vi "XLP80_EA_ReadStatus_Stack.vi"(8 "err in":errorcluster, 11 "Device information":string[](array[string])=["ASRL1::INSTR", "EL 3160-60 A", "000", "///", "1", "160", "60", "400", "10", "400"]) -> (0 "err out":errorcluster, 2 "Remote ON":bool, 3 "Device information IN":string[](array[string])=["ASRL1::INSTR", "EL 3160-60 A", "000", "///", "1", "160", "60", "400", "10", "400"])   [LabVIEW 2021]
uses:
  XLP80_EA_TDefsCluster_EA Feedback.ctl
  XLP80_EA_Globals.vi
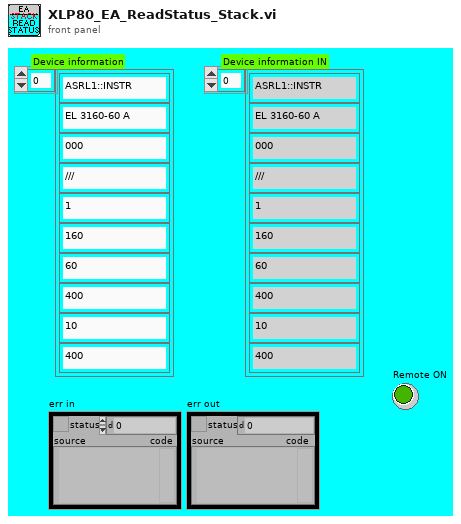
[diagram p1: front panel]
types:
  T1 = typedef "XLP80_EA_TDefsCluster_EA Feedback.ctl" = cluster{"EA on":bool, "Current":sgl, "Voltage":sgl, "Remote on":bool}
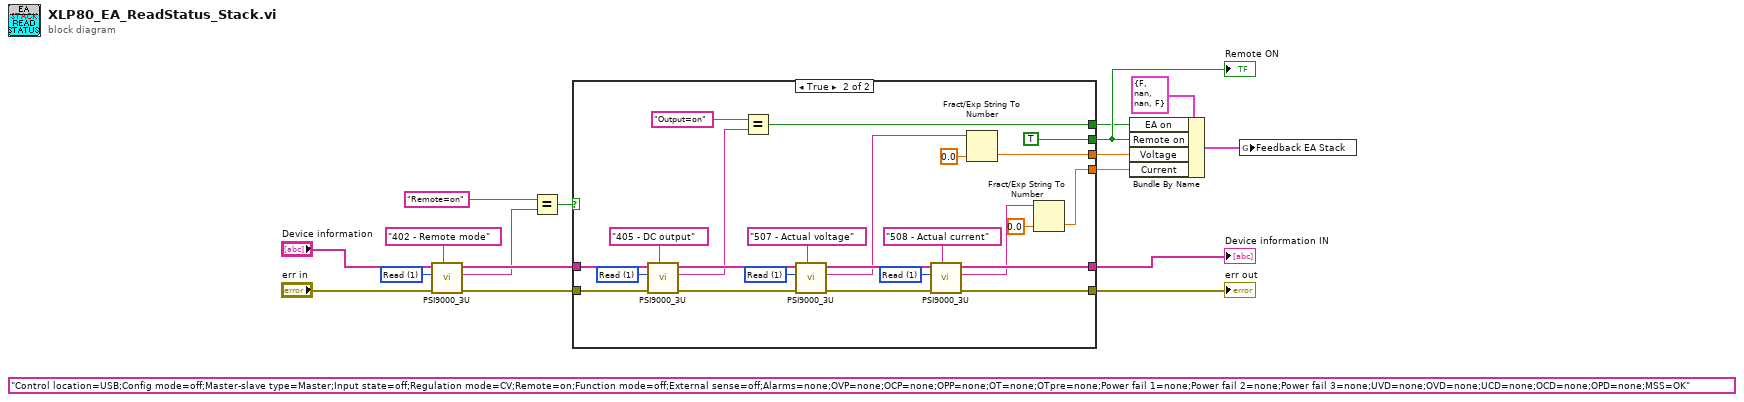
[diagram p0: block diagram]
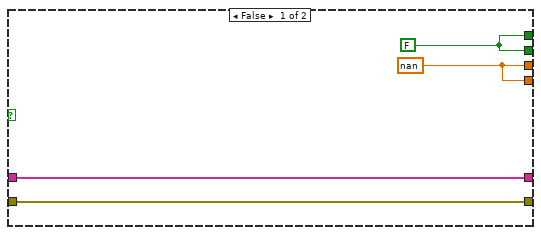
[diagram p2: hidden frame]
diagram:
  w12 = u8 1 items=["Write", "Read"] ("Access")
  (unwired) "Control location=USB;Config mode=off;Master-slave type=Master;Input state=off;Regulation mode=CV;Remote=on;Function mode=off;External sense=off;Alarms=none;OVP=none;OCP=none;OPP=none;OT=none;OTpre=none;Power fail 1=none;Power fail 2=none;Power fail 3=none;UVD=none;OVD=none;UCD=none;OCD=none;OPD=none;MSS=OK" ("Read data")
  n1 = call <instrlib>:"PSI9000_3U.vi"("Command list"="402 - Remote mode", "Error in"="err in", "Access"=w12, "Device information in"="Device information") -> ("Error out"=w10:errorcluster, "Read data"=w7:string, "Device information out"=w8:string[])  [unwired: 2 in, 1 out]
  n2 = Equal?(x="Remote=on", y=w7) -> (x = y?=w5:bool)
  n3 = case shown="True" w5 {
    tunnel: w8 -> [w20 w30]
    tunnel: w10 -> [w19 w32]
    tunnel: [w20 w41] -> w16
    tunnel: [w19 w40] -> w15
    tunnel: [w21 w37] -> w14
    tunnel: [w21 w34] -> w13
    tunnel: [w18 TRUE ("Remote on")] -> w4
    tunnel: [w18 w26] -> w3
    frame False {
      w21 = sgl nan
      w18 = FALSE ("Remote on")
    }
    frame True {
      w33 = u8 1 items=["Write", "Read"] ("Access")
      w44 = u8 1 items=["Write", "Read"] ("Access")
      w45 = u8 1 items=["Write", "Read"] ("Access")
      n4 = call <instrlib>:"PSI9000_3U.vi"("Command list"="405 - DC output", "Error in"=w32, "Access"=w33, "Device information in"=w30) -> ("Error out"=w31:errorcluster, "Read data"=w28:string, "Device information out"=w29:string[])  [unwired: 2 in, 1 out]
      n5 = Equal?(x="Output=on", y=w28) -> (x = y?=w26:bool)
      n6 = call <instrlib>:"PSI9000_3U.vi"("Command list"="507 - Actual voltage", "Error in"=w31, "Access"=w45, "Device information in"=w29) -> ("Error out"=w43:errorcluster, "Read data"=w39:string, "Device information out"=w42:string[])  [unwired: 2 in, 1 out]
      n7 = call <instrlib>:"PSI9000_3U.vi"("Command list"="508 - Actual current", "Error in"=w43, "Access"=w44, "Device information in"=w42) -> ("Error out"=w40:errorcluster, "Read data"=w35:string, "Device information out"=w41:string[])  [unwired: 2 in, 1 out]
      n8 = Fract/Exp String To Number(string=w39, default (0 dbl)=sgl 0.0 ("default (0 DBL)")) -> (number=w37:sgl)  [unwired: 2 in, 1 out]
      n9 = Fract/Exp String To Number(string=w35, default (0 dbl)=sgl 0.0 ("default (0 DBL)")) -> (number=w34:sgl)  [unwired: 2 in, 1 out]
    }
  }
  "err out" <- w15
  "Remote ON" <- w4
  "Device information IN" <- w16
  n10 = Bundle By Name(cluster=T1 {"EA on"=FALSE, "Current"=nan, "Voltage"=nan, "Remote on"=FALSE} ("Feedback EA Rekuperation"), "EA on"=w3, "Remote on"=w4, "Voltage"=w14, "Current"=w13) -> (w17:T1)
  n11 = global write "XLP80_EA_Globals.vi" "Feedback EA Stack"(w17) -> ()
